vi "FileConfigFromDTO.vi"(8 "error in (no error)":errorcluster, 11 "FileConfigDTO":T2={"rootFolder"="", "maxFileSize"=-1, "maxFileCount"=-1, "baseName"="", "extension"="", "delimiter"="", "calendarFolderTree"=FALSE}) -> (0 "error out":errorcluster, 3 "FileConfig":T1={"rootFolder"=path "", "maxFileSize"=-1, "maxFileCount"=-1, "baseName"="", "extension"="", "delimiter"="", "calendarFolderTree"=FALSE})   [LabVIEW 2026, in "Lumberjack.lvlib"]
uses:
  Lumberjack.lvlib
  TypeDefs/ConfigDTO/FileConfigDTO.ctl
  TypeDefs/FileConfig.ctl
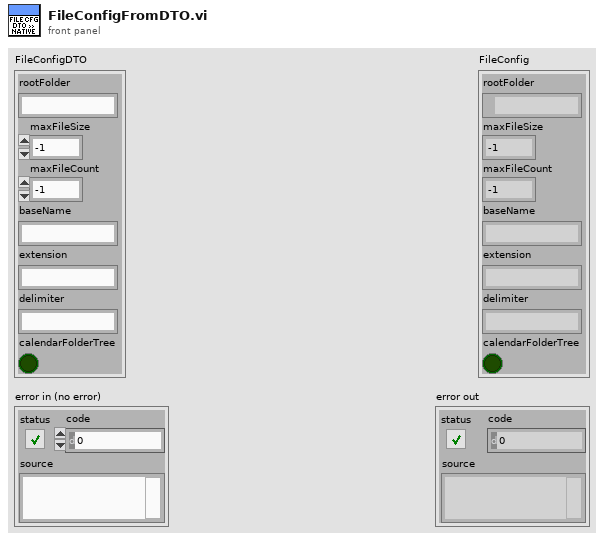
[diagram p1: front panel]
types:
  T1 = typedef "Lumberjack.lvlib/FileConfig.ctl" = cluster{"rootFolder":path, "maxFileSize":i64, "maxFileCount":i32, "baseName":string, "extension":string, "delimiter":string, "calendarFolderTree":bool}
  T2 = typedef "Lumberjack.lvlib/FileConfigDTO.ctl" = cluster{"rootFolder":string, "maxFileSize":i64, "maxFileCount":i32, "baseName":string, "extension":string, "delimiter":string, "calendarFolderTree":bool}
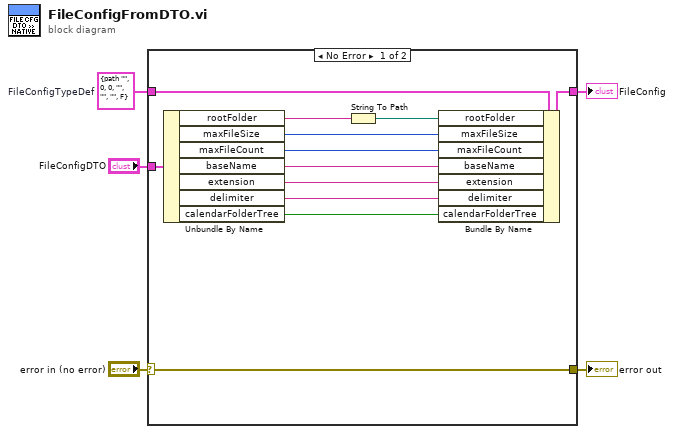
[diagram p0: block diagram]
diagram:
  w5 = T1 {"rootFolder"=path "", "maxFileSize"=0, "maxFileCount"=0, "baseName"="", "extension"="", "delimiter"="", "calendarFolderTree"=FALSE}  # FileConfigTypeDef
  n1 = case shown="No Error" "error in (no error)" {
    selector: "error in (no error)" -> [w6 w19]
    tunnel: [w6 w19] -> w1
    tunnel: "FileConfigDTO" -> [w16 _]
    tunnel: [w17 w18] -> w2
    tunnel: w5 -> [w15 w18]
    frame No Error {
      n2 = Unbundle By Name(w16) -> ("rootFolder"=w8:string, "maxFileSize"=w14:i64, "maxFileCount"=w13:i32, "baseName"=w12:string, "extension"=w11:string, "delimiter"=w10:string, "calendarFolderTree"=w9:bool)
      n3 = String To Path(string=w8) -> (path=w7:path)
      n4 = Bundle By Name(cluster=w15, "rootFolder"=w7, "maxFileSize"=w14, "maxFileCount"=w13, "baseName"=w12, "extension"=w11, "delimiter"=w10, "calendarFolderTree"=w9) -> (w17:T1)
    }
    frame Error {
    }
  }
  "error out" <- w1
  "FileConfig" <- w2
